vi "Report.vi"(6 "文件重命名":bool, 7 "文件名称":string, 8 "错误输入（无错误）":errorcluster, 10 "工位名称":string, 11 "判定结果":bool[][](array[boolean])=[[TRUE]]) -> (0 "error out":errorcluster caption="错误输出", 3 "RESULT_VALUE":string)   [LabVIEW 2020]
uses:
  Global_Variable/Global.vi
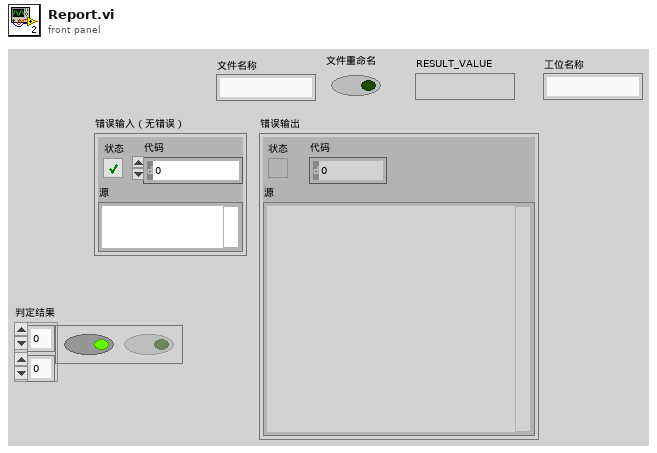
[diagram p1: front panel]
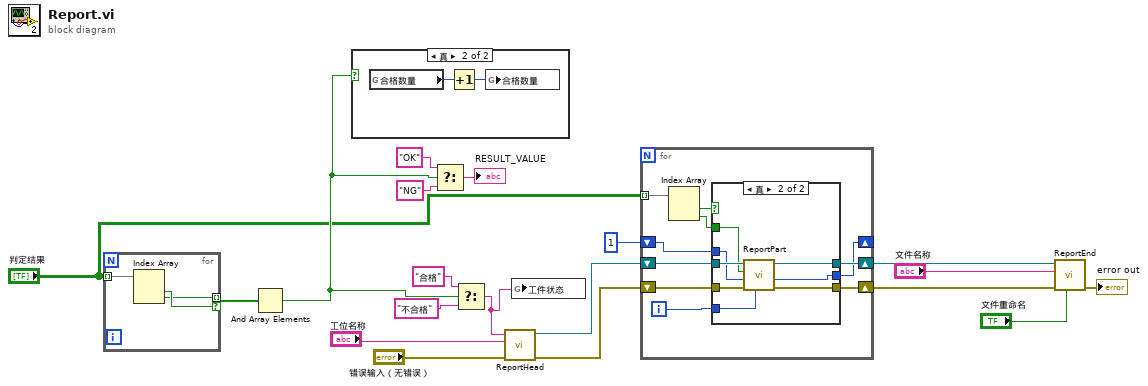
[diagram p0: block diagram]
diagram:
  n1 = for {
    tunnel: [w20] -> w7 mode=indexing if=w21
    tunnel: "判定结果" -> [w22] mode=indexing
    n2 = Index Array(array=w22) -> (element #1=w21:bool, element #2=w20:bool)  [unwired: 2 in]
  }
  n3 = And Array Elements(Boolean array=w7) -> (logical AND=w6:bool)
  n4 = case shown="真" w6 {
    frame False {
    }
    frame True {
      n5 = global read "Global.vi" "合格数量"() -> (w23:i32)
      n6 = Increment(x=w23) -> (x+1=w24:i32)
      n7 = global write "Global.vi" "合格数量"(w24) -> ()
    }
  }
  n8 = Select(t="OK", s=w6, f="NG") -> (s? t:f=→"RESULT_VALUE":string)
  n9 = Select(t="合格", s=w6, f="不合格") -> (s? t:f=w2:string)
  n10 = call "ReportHead.vi"("error in (no error)"="错误输入（无错误）", "工位名称"="工位名称", "产品状态"=w2) -> ("error out"=w18:errorcluster, "report out"=w19:refnum<class "NI_report.lvclass">)  [unwired: 7 in]
  n11 = global write "追溯全部变量.vi" "工件状态"(w2) -> ()
  n12 = for {
    shift-right: [w32] -> w17
    shift-left: w19 -> [w34]
    shift-right: [w31] -> w16
    shift-left: w18 -> [w33]
    tunnel: "判定结果" -> [w27] mode=indexing
    shift-right: [w28] -> _
    shift-left: 1 ("索引") -> [w29]
    i -> [w30]
    n13 = Index Array(array=w27) -> (element #1=w26:bool, element #2=w25:bool)  [unwired: 2 in]
    n14 = case shown="真" w26 {
      tunnel: w34 -> [w36 w45]
      tunnel: w33 -> [w37 w44]
      tunnel: [w36 w43] -> w32
      tunnel: [w37 w42] -> w31
      tunnel: w30 -> [_ w39]
      tunnel: w29 -> [w35 w41]
      tunnel: [w35 w40] -> w28
      tunnel: w25 -> [_ w38]
      frame False {
      }
      frame True {
        n15 = call "ReportPart.vi"("试验项目"=w39, "error in"=w44, "索引"=w41, "合格"=w38, "report in"=w45) -> ("error out 2"=w42:errorcluster, "索引OUT"=w40:i32, "report out"=w43:refnum<class "NI_report.lvclass">)  [unwired: 4 in]
      }
    }
  }
  n16 = call "ReportEnd.vi"("文件重命名"="文件重命名", "error in (no error)"=w16, "文件名称"="文件名称", "report in"=w17) -> ("error out"=→"error out":errorcluster)  [unwired: 7 in]
